vi "10.4.vi"() -> ()   [LabVIEW 2019]
panel:
  in  "stop":bool
  out "2":dbl(graph)
  out "1":dbl(graph)
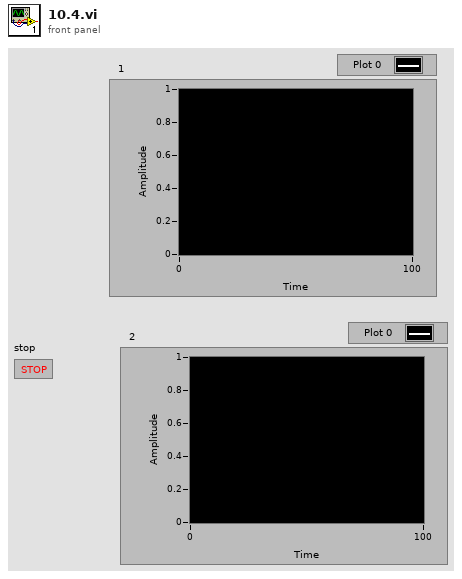
[diagram p1: front panel]
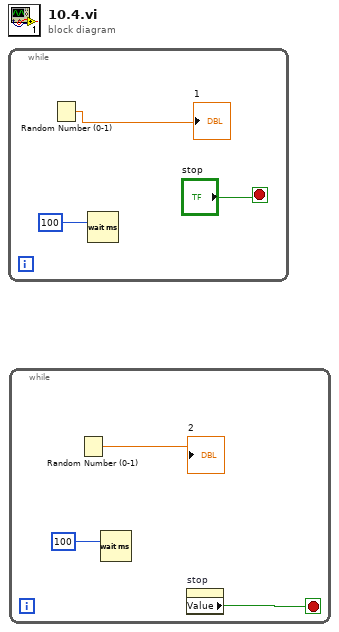
[diagram p0: block diagram]
diagram:
  n1 = while {
    stop <- "stop" stop-if-true
    n2 = Random Number (0-1)() -> (number: 0 to 1=→"1":dbl)
    n3 = Wait (ms)(milliseconds to wait=100) -> ()  [unwired: 1 out]
  }
  n4 = while {
    stop <- w5 stop-if-true
    n5 = Random Number (0-1)() -> (number: 0 to 1=→"2":dbl)
    n6 = Wait (ms)(milliseconds to wait=100) -> ()  [unwired: 1 out]
    n7 = property on="stop" class="Bool (strict)"() -> ("Value"=w5:bool)  [unwired: 2 in, 2 out]
  }
